vi "Write Connected Port.vi"(8 "error in (no error)":errorcluster, 10 "Connected Port":u16, 11 "ReceiverState in":refnum<class "Connect Command.lvclass">) -> (0 "error out":errorcluster, 3 "ReceiverState out":refnum<class "Connect Command.lvclass">)   [LabVIEW 2013, in "Receiver.lvlib" / "Receive Commands Using State Actors.lvlib" / "Connect Command.lvlib" / "Connect Command.lvclass"]
uses:
  Connect Command/Connect Command.lvclass
  Connect Command/Connect Command.lvclass/Connect Command.ctl
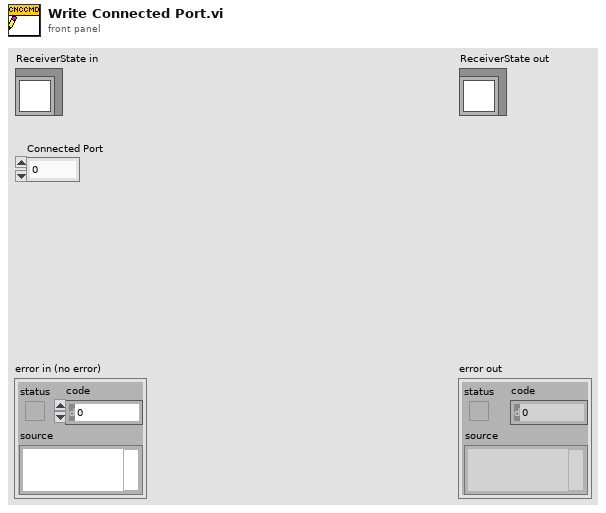
[diagram p1: front panel]
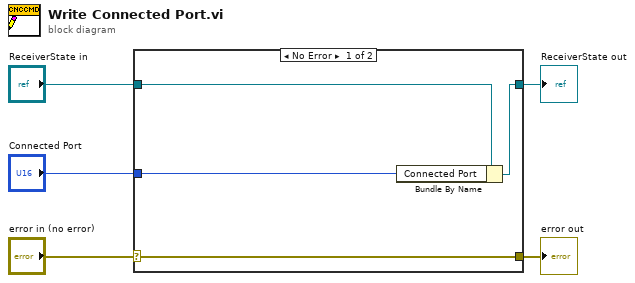
[diagram p0: block diagram]
diagram:
  n1 = case shown="No Error" "error in (no error)" {
    selector: "error in (no error)" -> [w9 w10]
    tunnel: [w9 w10] -> w4
    tunnel: [w7 w11] -> w2
    tunnel: "ReceiverState in" -> [w8 w11]
    tunnel: "Connected Port" -> [w6 _]
    frame No Error {
      n2 = Bundle By Name(cluster=w8, "Connected Port"=w6) -> (w7:refnum<class "Connect Command.lvclass">)
    }
    frame Error {
    }
  }
  "error out" <- w4
  "ReceiverState out" <- w2
